vi "IETS_Tool_14_ProbeStation_SweepSaver.vi"() -> ()   [LabVIEW 2013]
doc: "I. Description:\nThis example demonstrates how to continuously acquire and generate data at the same time, synchronized with one another.\n\nII. Instructions for Running:\n1. Select the physical channel to correspond to where your signal is input on the DAQ device. Also, select the corresponding channel for where your signal is being generated.\n2. Enter the minimum and maximum voltage ranges.\nNote: For better accuracy try to match the input range to the expected voltage level of the measured signal.\n3. Set the sample rate of the acquisition.\nNote: The rate should be at least twice as fast as the maximum frequency component of the signal being acquired. \n6. Select the Rate for the generation\n7. Select what type of signal to generate and the amplitude.\nNote: This example requires two DMA channels to run. If your hardware does not support two DMA channels, you need to set the Data Transfer Mechanism property for the Analog Output Task to use \"Interrupts\". The Data Transfer Mechanism property is located in the DAQmx Channel Property hierarchy at:\n\nDAQmx Channel Property Node>>Analog Output>>General Properties>>Advanced>>Data Transfer and Memory>>Data Transfer Mechanism\n\nRefer to your device documentation to determine how many DMA channels are supported for your hardware.\n\nIII. Block Diagram Steps:\n1. Create an analog input voltage channel. Also, create an analog output voltage channel.\n2. Set the rate for the sample clock. Additionally, define the sample mode to be continuous. Also, set the sample clock rate for the signal generation.\n2a. Call the Get Terminal Name with Device Prefix VI. This will take a Task and a terminal and create a properly formatted device + terminal name to use as the source of the Trigger.\n3. Define the parameters for a Digital Edge Start Trigger. Set the Analog output to trigger off the AI Start Trigger. This is an internal trigger signal.\n4. Use the Basic Function Generator VI to create the signal to be generated.\n5. Call the Start VI to arm the two functions. Make sure the analog output is armed before the analog input. This will ensure both will start at the same time.\n6. Read the waveform data in a loop until the user hits the stop button or an error occurs. The Is Task Done? VI is used to check for errors in the Analog Output Task.\n7. Call the Clear VI to Clear the Task\n8. Use the popup dialog box to display an error if any.\n\nIV. I/O Connections Overview:\nMake sure your signal input/output terminals match the Physical Channel I/O controls."
uses:
  <vilib>/Utility/error.llb/DialogType.ctl
  <vilib>/DAQmx/write.llb/DAQmx Write (Analog 2D DBL NChan NSamp).vi
  <vilib>/DAQmx/read.llb/DAQmx Read (Analog 1D DBL NChan 1Samp).vi
  <vilib>/DAQmx/write.llb/DAQmx Write (Analog DBL 1Chan 1Samp).vi
  <vilib>/DAQmx/read.llb/DAQmx Read (Analog DBL 1Chan 1Samp).vi
  <vilib>/Analysis/baseanly.llb/Mean (DBL).vi
  <vilib>/DAQmx/write.llb/DAQmx Write (Analog 1D DBL NChan 1Samp).vi
  <vilib>/DAQmx/create/channels.llb/DAQmx Create Channel (AO-Voltage-Basic).vi
  <vilib>/DAQmx/create/channels.llb/DAQmx Create Channel (AI-Voltage-Basic).vi
  <vilib>/DAQmx/configure/timing.llb/DAQmx Timing (Sample Clock).vi
  <vilib>/DAQmx/configure/trigger.llb/DAQmx Start Trigger (Digital Edge).vi
  <vilib>/DAQmx/miscellaneous.llb/DAQmx Fill In Error Info.vi
  <vilib>/Utility/file.llb/Write To Spreadsheet File (DBL).vi
  pid/pid.llb/PID (DBL).vi
  pid/pid.llb/PID Output Rate Limiter (DBL).vi
  <vilib>/ptbypt/NI_PtbyPt.lvlib
  <resource>/objmgr/daqmx.rc
  <vilib>/Analysis/NI_AALBase.lvlib
panel:
  in  "Bias Offset Correct":dbl
  out "Bias Sweep":dbl[](graph)
  out "element":dbl
  out "mean":dbl format="%.6f"
  out "size(s)":i32
  out "Numeric":i32
  in  "PID":bool=TRUE caption="Step Z"
  in  "Tab Control":enum32{"PID Controller", "Tapping Controls"}(tab)=enum."Tapping Controls"
  in  "Proportional Gain":dbl=0.0001
  in  "Integral Gain":dbl=1e-07
  in  "Differential Gain":dbl=1e-05
  in  "Setpoint":dbl=0.1
  in  "Piezo Delta rate":dbl=1000.0
  in  "Min Current":dbl=0.002
  in  "Max Current":dbl=10.2
  in  "Ramp Rate":dbl=20.0
  in  "Make Contact":i32=1200
  in  "Break Contact":i32=500
  in  "Step Length":i32=100
  in  "Step Max":dbl=0.3
  in  "Step Min":dbl=0.05
  out "Tapping Stop":bool
  out "Case":i32
  in  "Contact Cycles":i32
  in  "Tapping":bool caption="Step Z"
  out "x/y":dbl
  out "Waveform Chart":dbl(graph)
  in  "Analog Ouyput 1":dbl(slide) min=-10.0 max=10.0 step=0.001 scale=-10.0..10.0
  in  "Manual Z":bool caption="Step Z"
  in  "Sweep Amplitude":dbl=1.0
  in  "Stop Sweep":bool
  out "Connections 2":string="AI0=Current\nAI1=Bias\nAI2=dI/dV\nAI3=d2I/dV2\nAI4=X-Axis\nAI5=Z-Axis\n"
  out "Connections":string="AO0=Bias\nAO1=Z-axis\nAO2=X-Axis\nAO3=NA"
  out "Save Indicator":bool
  in  "Z-Direction":bool caption="Step Z"
  in  "Update Bias":bool
  in  "Save Decay":bool
  in  "Step Z":bool
  in  "Comment":string="Molecule=TP4\nGain=10nA\nBias Gain=div/1\nSweep Freq.=0.0008Hz\nRef. Bias=4mV\nRef. Freq=2.977kHz\nGain LIA1=2mV\nTC LIA1=1s\nGain LIA2=5mV\nTC LIA2=1s\nLIA1=EGG\nLIA2=SRS\nEGG is driving(possible 5mV offset)"
  in  "Filenumber":i32
  in  "DATA Filename":string="Data_"
  in  "Data Directory":path=path "E:/Research/Data"
  out "Current Decay":cluster{dbl[], dbl[]}(graph)
  out "d2I/dV2":cluster{dbl[], dbl[]}(graph)
  out "dI/dV":cluster{dbl[], dbl[]}(graph)
  out "IV":cluster{dbl[], dbl[]}(graph)
  in  "# Samples":i32=2000
  in  "Frequency (Hz)":dbl=1.0
  out "Measurement 2":cluster{i32, dbl, dbl[]}(graph) caption="Measurement"
  out "Actual Update Generation Rate 2":dbl=5000.0 caption="Actual Update Generation Rate" format="%0.2f"
  in  "stop 3":bool
  in  "Bias":dbl=0.1 caption="Bias Start Point" step=0.1 format="%_3g"
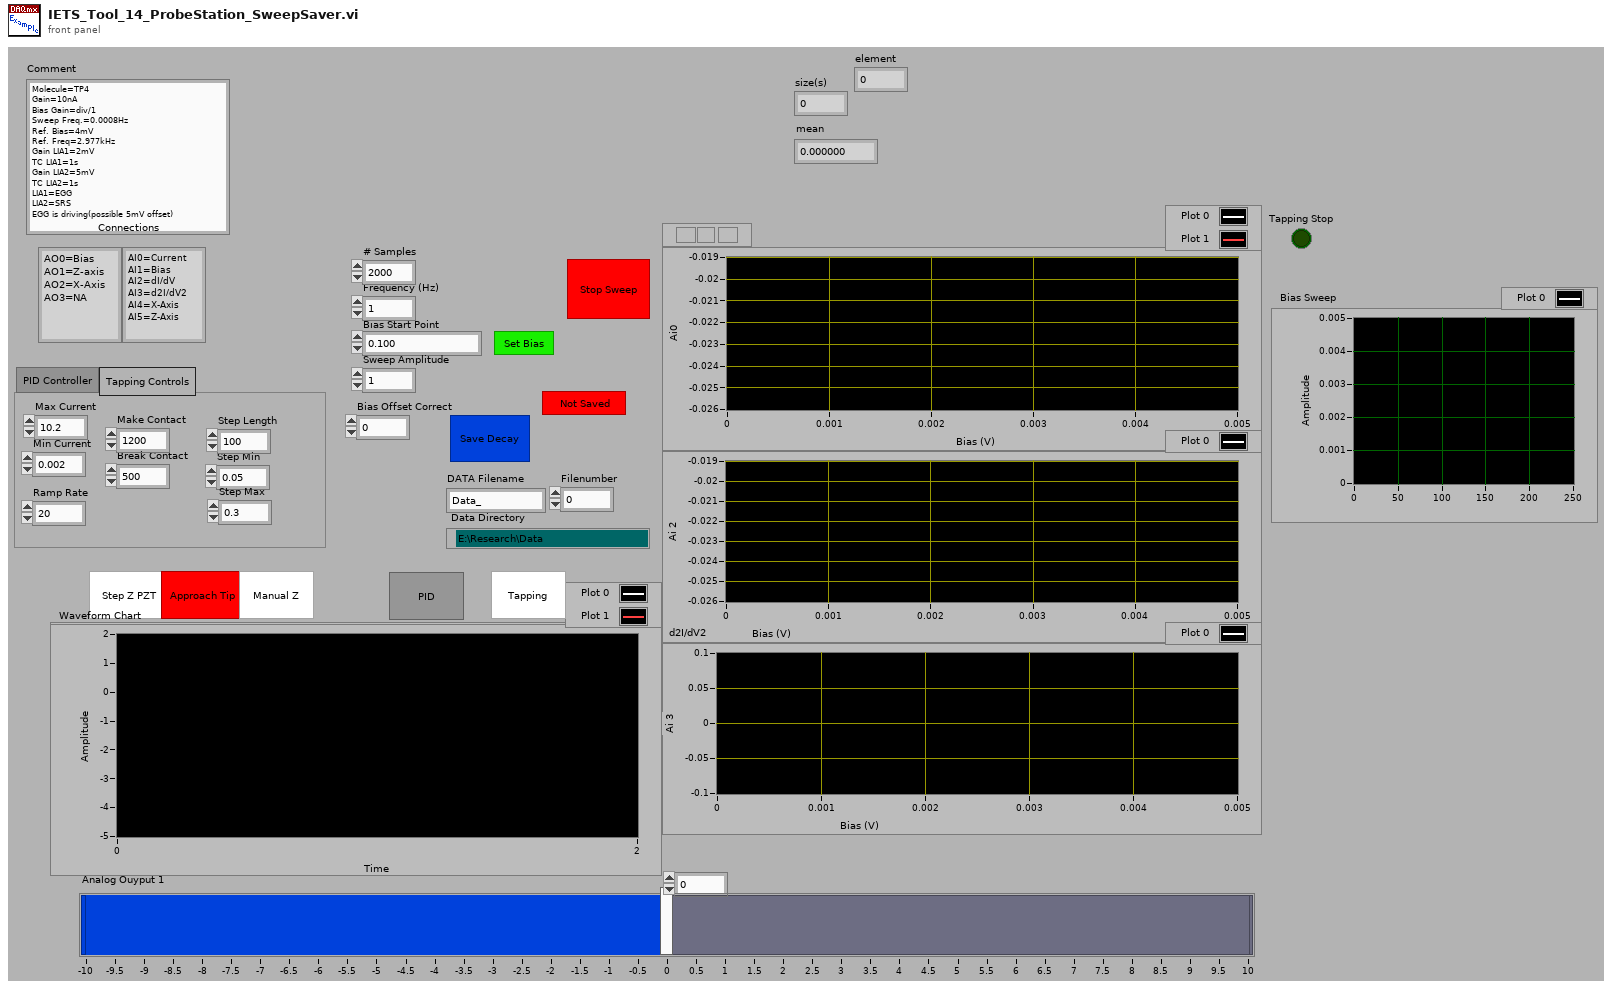
[diagram p1: front panel]
types:
  T1 = enum16{"open", "replace", "create", "open or create", "replace or create", "replace or create with confirmation"}
  T2 = typedef "DialogType.ctl" = u16
  T3 = cluster{"Proportional Gain":dbl, "Integral Gain ":dbl, "Differential Gain":dbl}
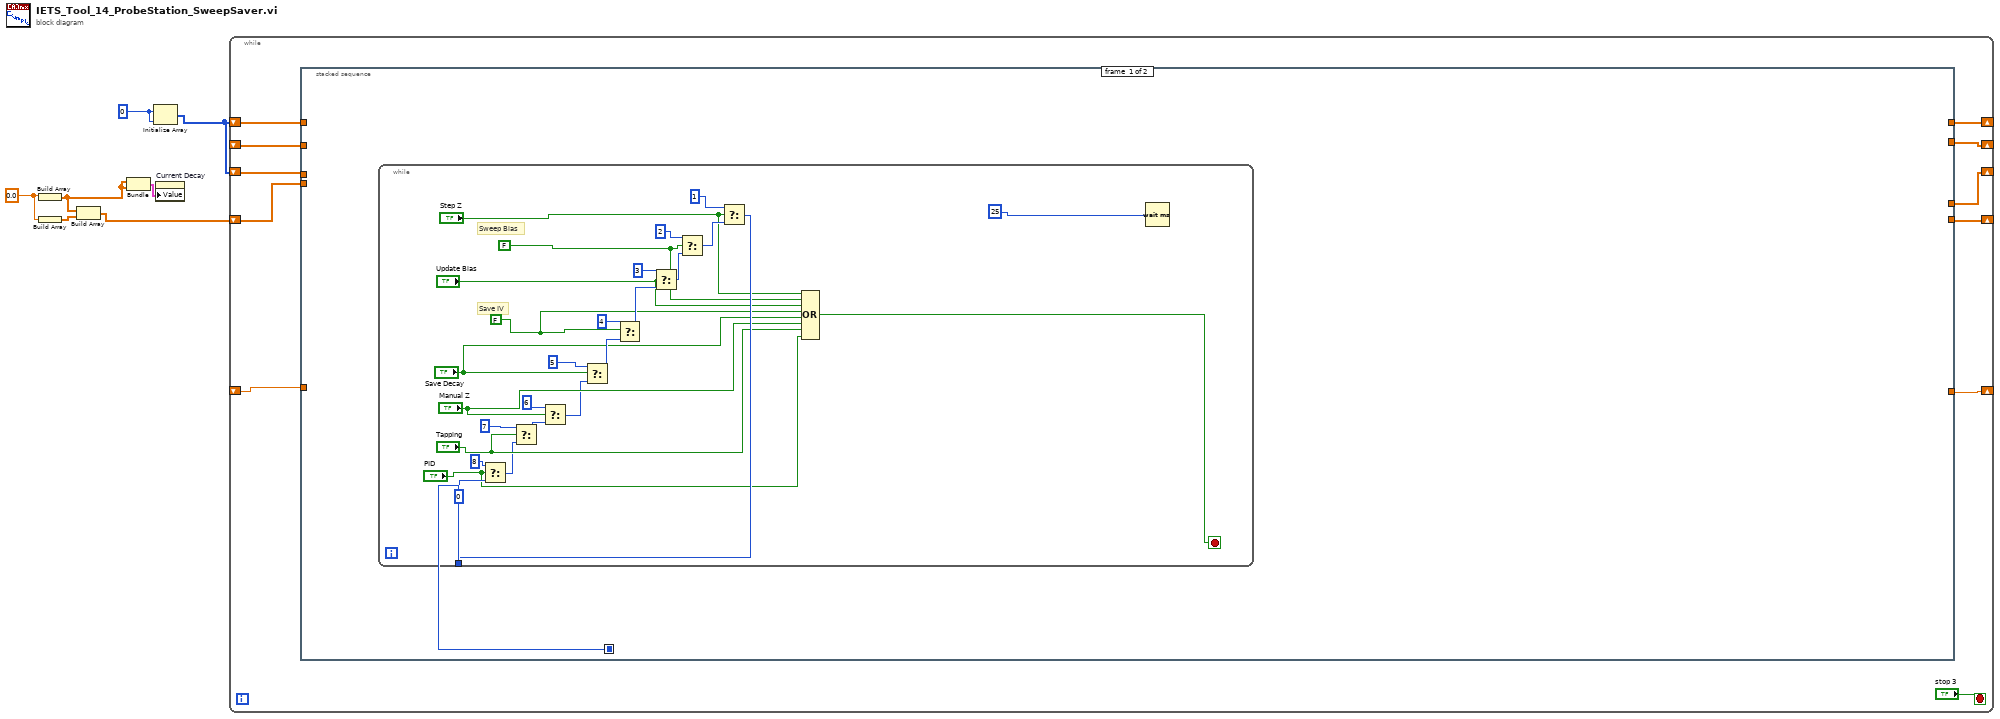
[diagram p0: block diagram]
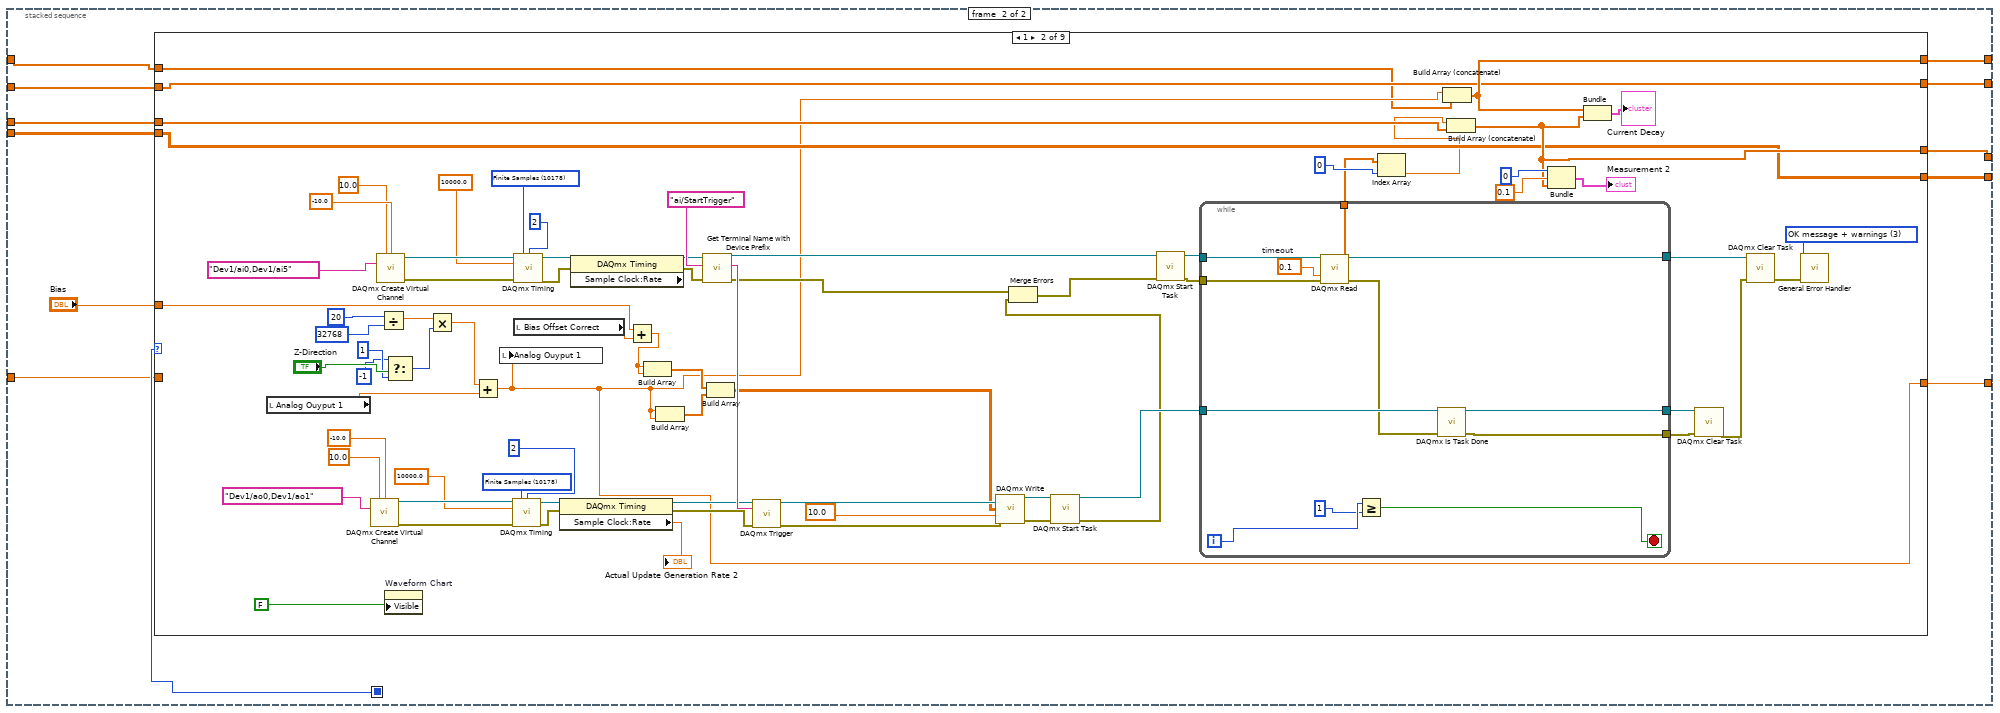
[diagram p2: hidden frame]
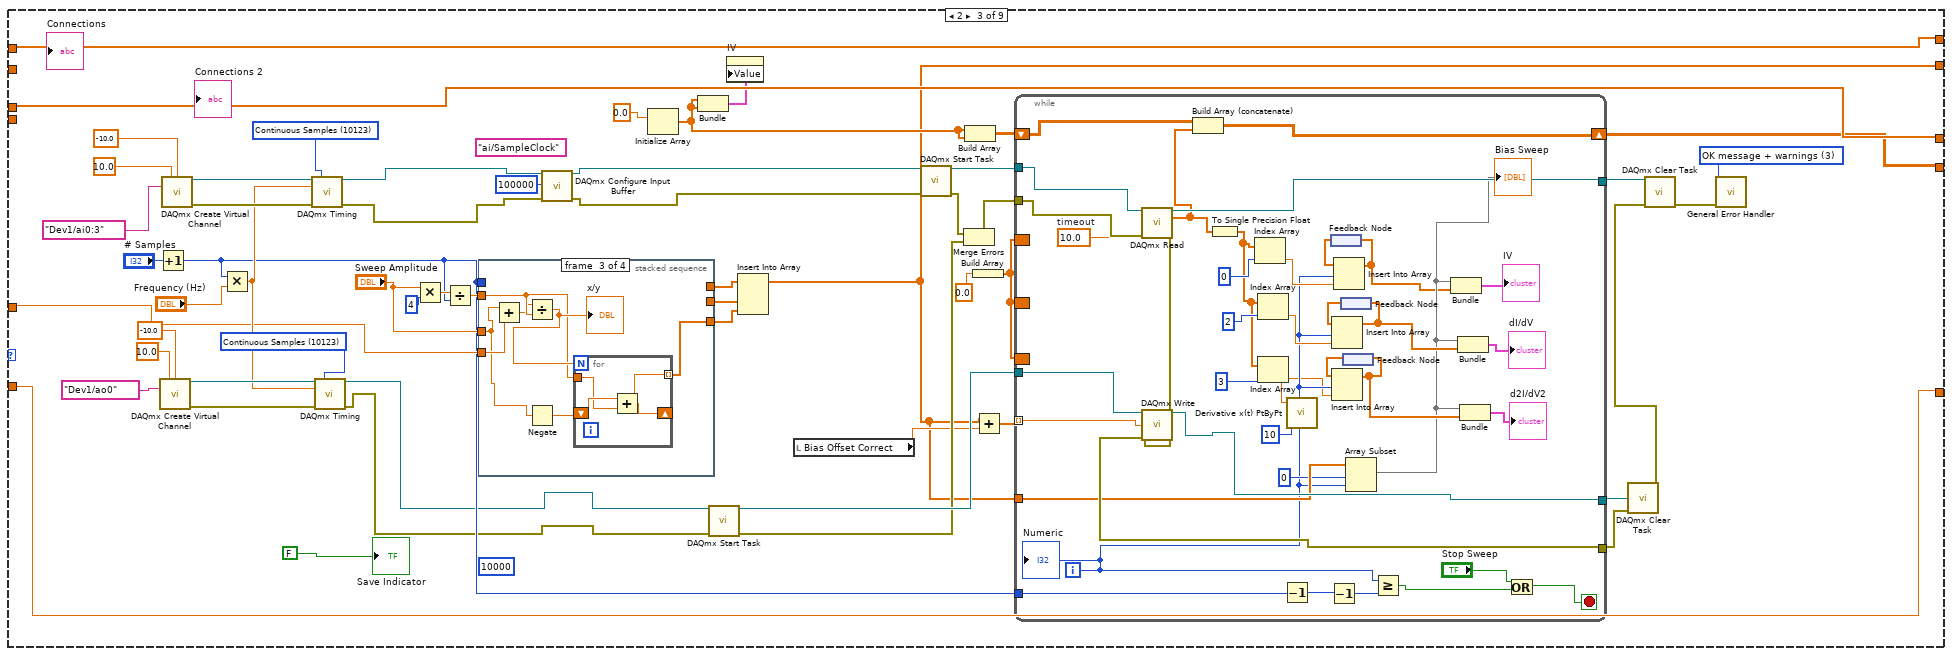
[diagram p4: hidden frame]
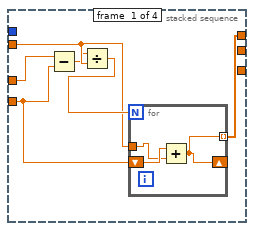
[diagram p5: hidden frame]
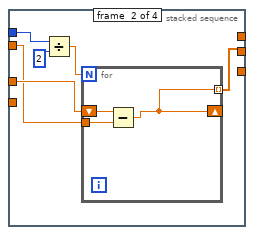
[diagram p6: hidden frame]
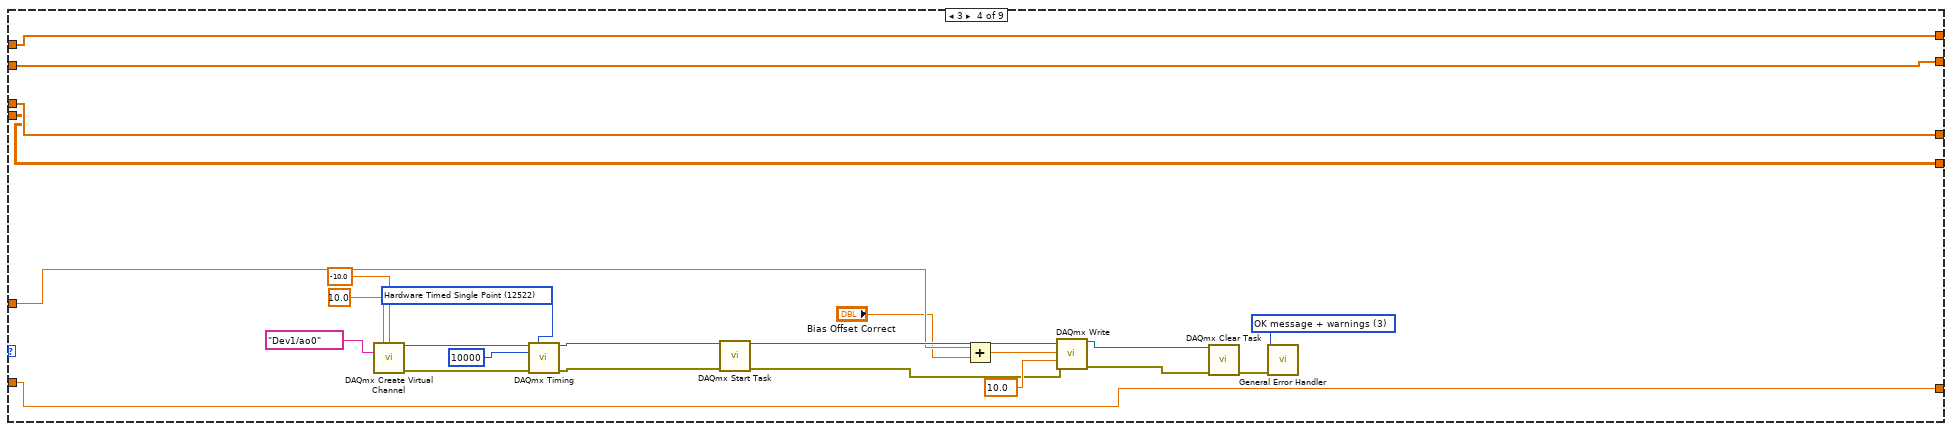
[diagram p8: hidden frame]
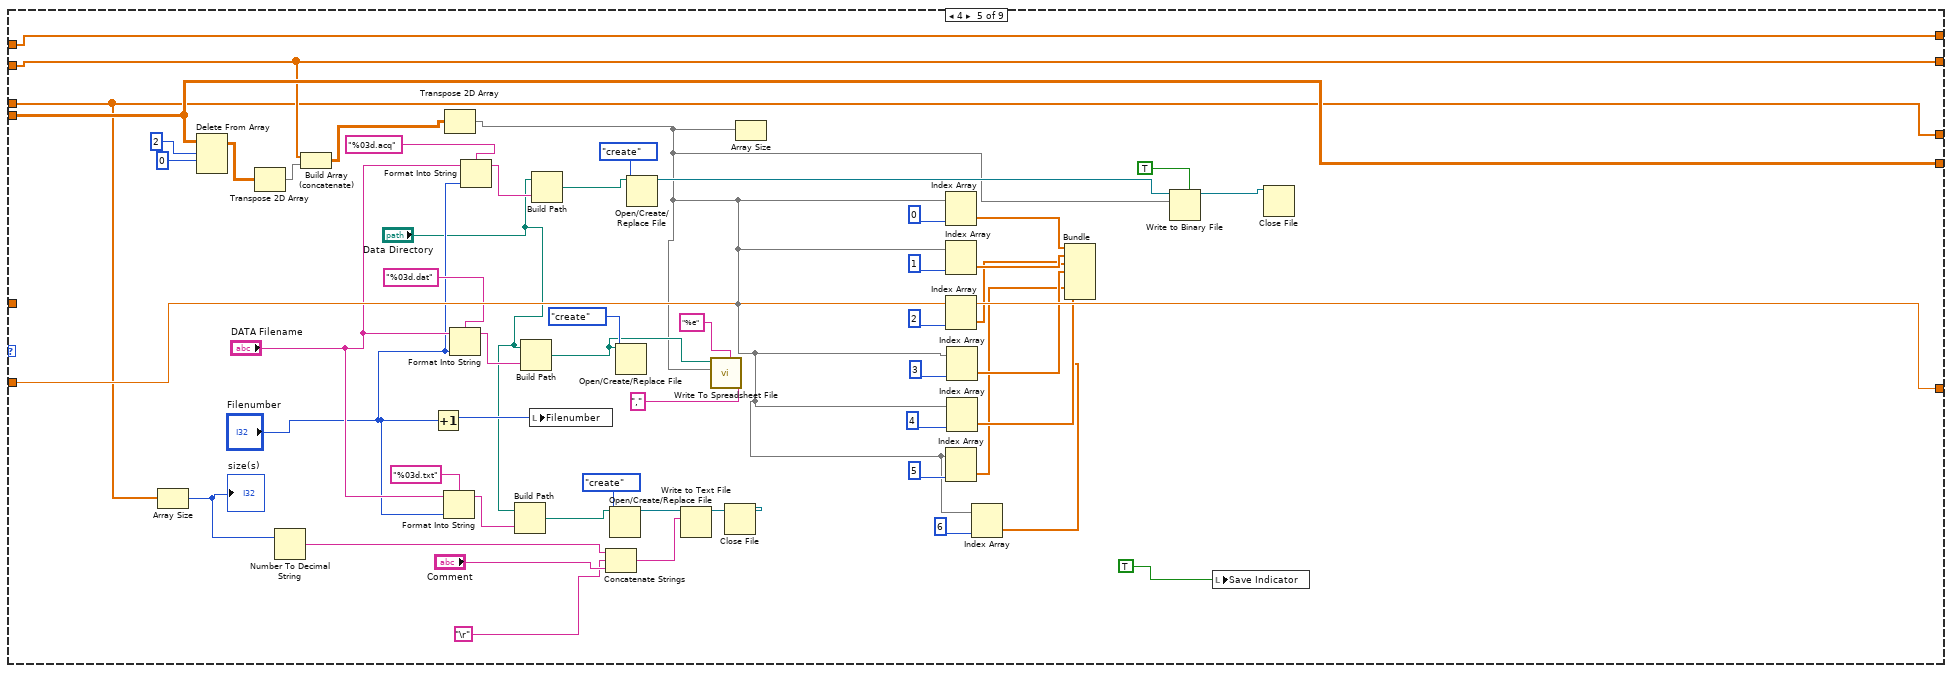
[diagram p9: hidden frame]
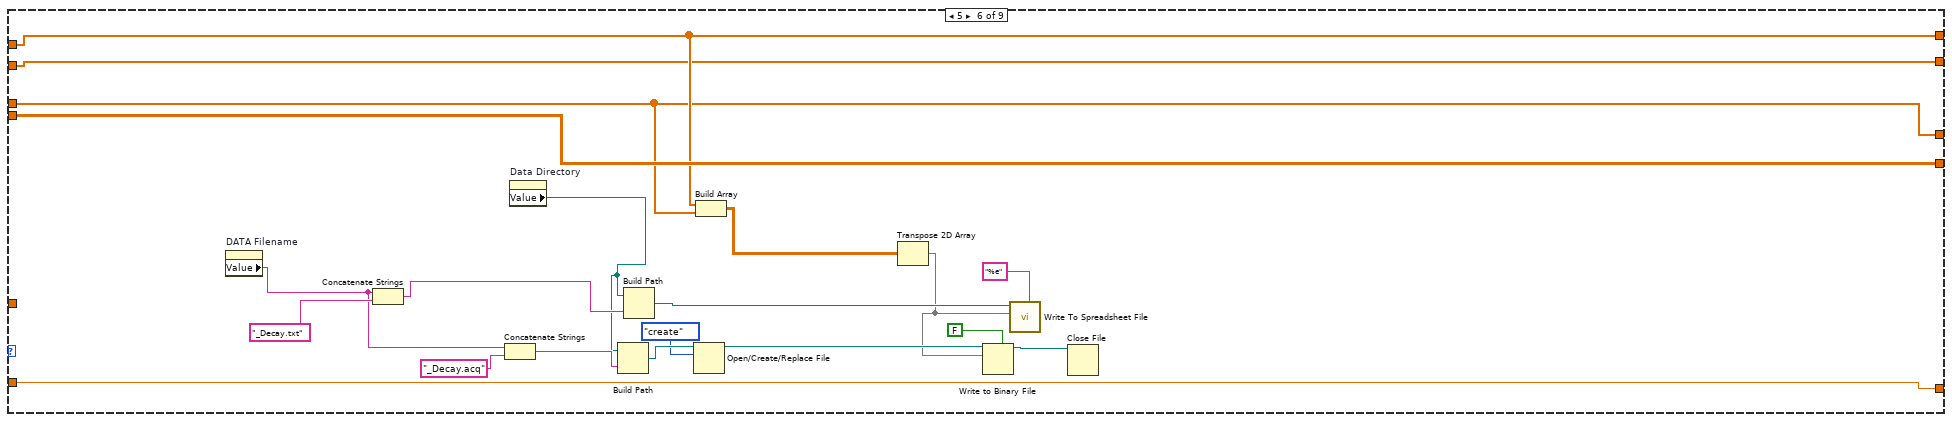
[diagram p10: hidden frame]
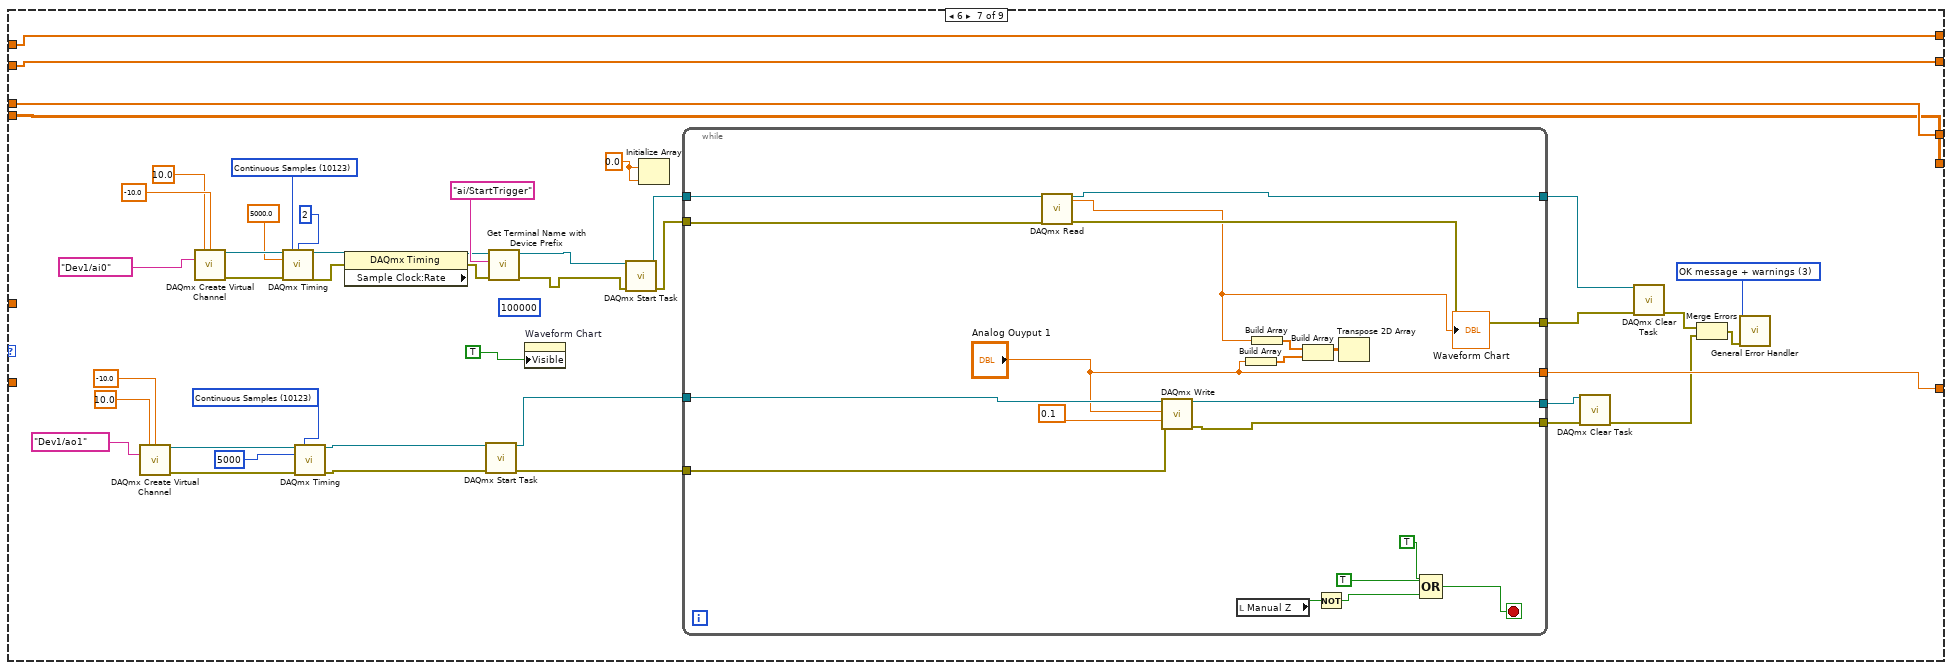
[diagram p11: hidden frame]
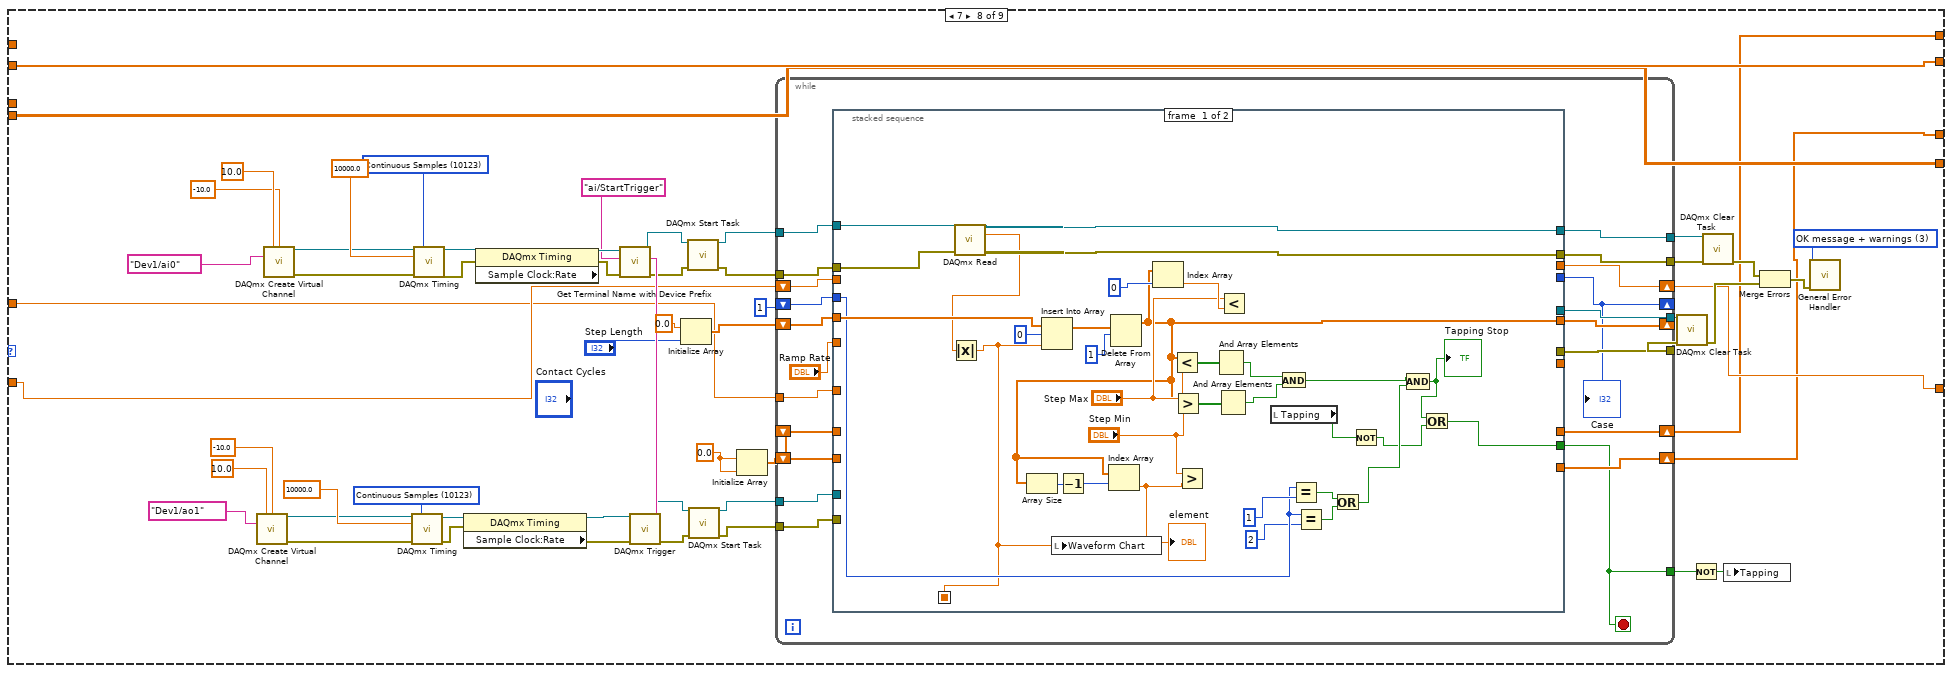
[diagram p12: hidden frame]
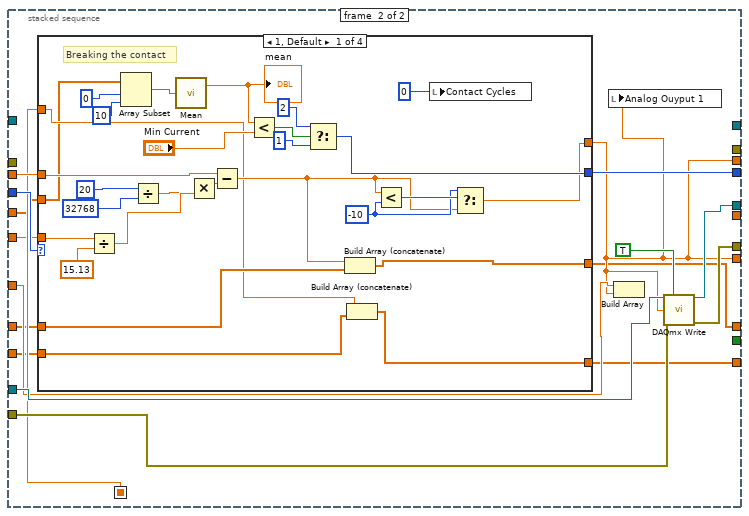
[diagram p13: hidden frame]
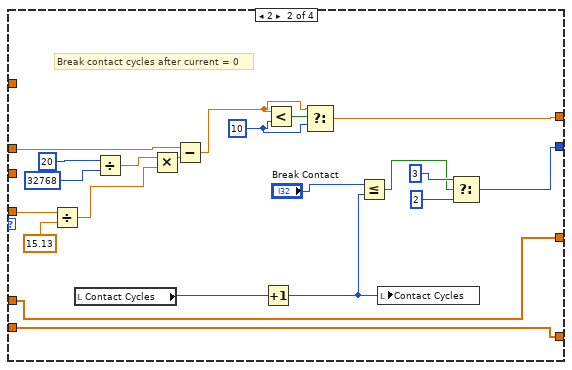
[diagram p14: hidden frame]
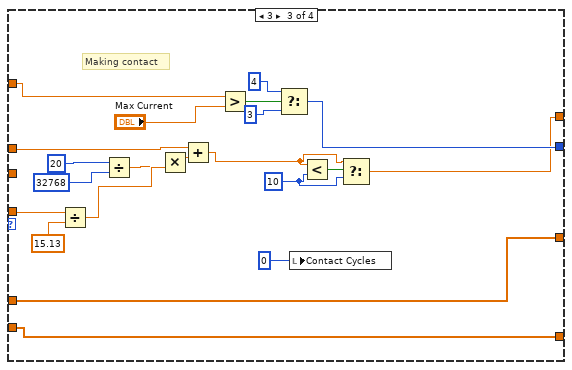
[diagram p15: hidden frame]
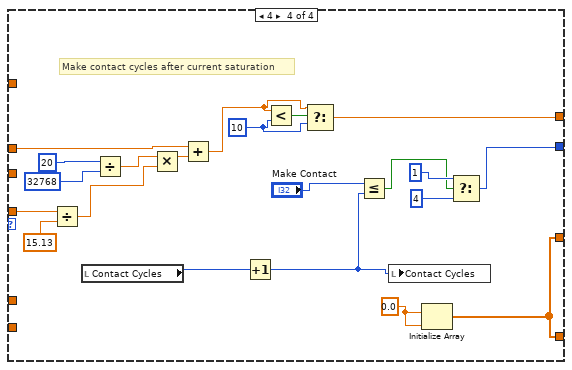
[diagram p16: hidden frame]
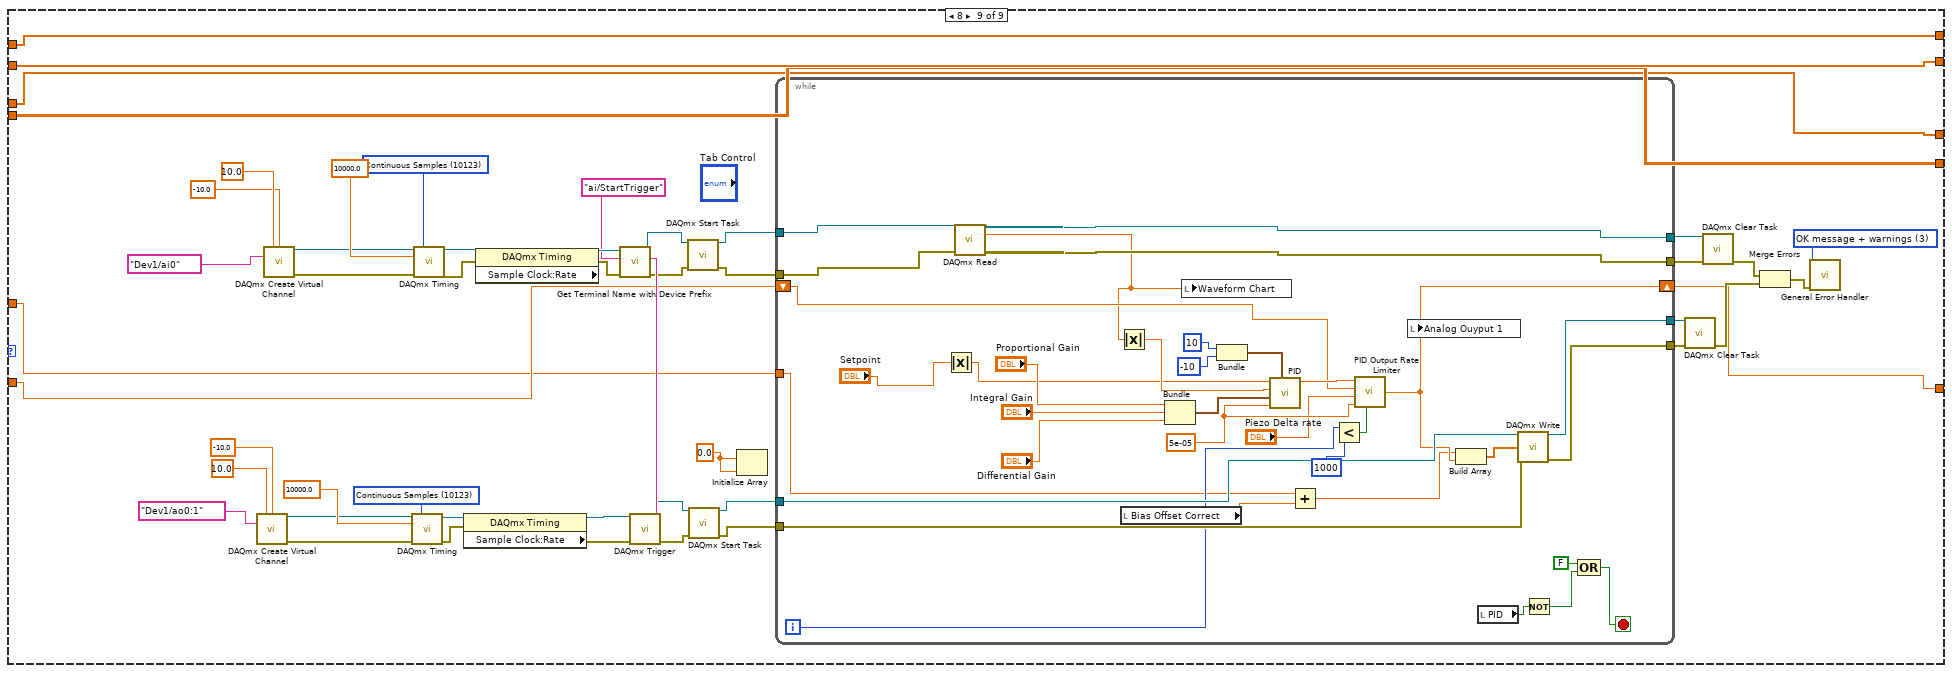
[diagram p17: hidden frame]
diagram:
  w2 = 0
  w7 = 0.0
  n1 = Build Array(w7) -> (w4:dbl[])
  n2 = Build Array(w7) -> (w6:dbl[])
  n3 = Build Array(w4, w6) -> (w5:dbl[][])
  n4 = Bundle(w4, w4) -> (w3:cluster{dbl[], dbl[]})  [unwired: 1 in]
  n5 = Initialize Array(w2, w2) -> (w1:i32[])
  n6 = property on="Current Decay" class="XYGraph (strict)"("Value"=w3) -> ()  [unwired: 2 in, 2 out]
  n7 = while {
    shift-right: [w16] -> _
    shift-left: w1 -> [w17]
    shift-right: [w14] -> _
    shift-left: w1 -> [w15]
    shift-right: [w12] -> _
    shift-left: _ -> [w13]
    shift-right: [w10] -> _
    shift-left: w5 -> [w11]
    shift-right: [w8] -> _
    shift-left: _ -> [w9]
    stop <- "stop 3" stop-if-true
    n8 = stacked-sequence {
      seq-local: [w19 _] -> [_ w58]
      tunnel: w17 -> [_ w57]
      tunnel: [_ w56] -> w16
      tunnel: w15 -> [_ w54]
      tunnel: [_ w53] -> w14
      tunnel: w13 -> [_ w52]
      tunnel: [_ w47] -> w12
      tunnel: w11 -> [_ w51]
      tunnel: [_ w50] -> w10
      tunnel: w9 -> [_ w49]
      tunnel: [_ w48] -> w8
      frame #0 {
        n9 = while {
          tunnel: [w37] -> w19
          stop <- w36 stop-if-true
          w20 = FALSE ("Sweep Bias")
          w21 = FALSE ("Save IV")
          # "Sweep Bias"
          # "Save IV"
          n10 = Select(t=8, s="PID", f=0) -> (s? t:f=w25:i32)
          n11 = Select(t=7, s="Tapping", f=w25) -> (s? t:f=w27:i32)
          n12 = Select(t=6, s="Manual Z", f=w27) -> (s? t:f=w28:i32)
          n13 = Select(t=5, s="Save Decay", f=w28) -> (s? t:f=w42:i32)
          n14 = Select(t=4, s=w21, f=w42) -> (s? t:f=w41:i32)
          n15 = Select(t=3, s="Update Bias", f=w41) -> (s? t:f=w39:i32)
          n16 = Select(t=2, s=w20, f=w39) -> (s? t:f=w46:i32)
          n17 = Select(t=1, s="Step Z", f=w46) -> (s? t:f=w37:i32)
          n18 = Compound Arithmetic op=OR("Step Z", w20, "Update Bias", w21, "Save Decay", "Manual Z", "Tapping", "PID") -> (w36:bool)
          n19 = Wait (ms)(milliseconds to wait=25) -> ()  [unwired: 1 out]
        }
      }
      frame #1 {
        n20 = case shown="1" w58 {
          tunnel: w57 -> [w63 w70 w190 w281 w301 w367 w412 _ w652]
          tunnel: [w63 w83 w190 w281 w301 w367 w412 w438 w652] -> w56
          tunnel: "Bias" -> [_ w66 w175 w275 _ _ _ w444 w651]
          tunnel: w54 -> [w62 w67 w187 w282 w347 w368 w414 _ w653]
          tunnel: [w62 w84 w187 w282 w347 w368 w414 w439 w653] -> w53
          tunnel: w52 -> [w61 _ w186 w280 w346 w369 _ w445 w660]
          tunnel: [w61 w68 w186 w280 w346 w369 w383 w440 w657] -> w47
          tunnel: w51 -> [w60 w81 _ w278 w326 w370 w411 w442 w658]
          tunnel: [w60 w81 w167 w278 w326 w370 w411 w442 w658] -> w50
          tunnel: [w59 w76 w151 w277 w324 w352 w413 w443 w659] -> w48
          tunnel: w49 -> [w59 w76 _ w277 w324 w352 w413 w443 w659]
          frame 0, Default {
          }
          frame 1 {
            w118 = T2 3 items=["no dialog", "OK message", "continue or stop message", "OK message + warnings", "continue/stop + warnings"] ("type of dialog (OK msg:1)")
            w130 = 10178 items=["Finite Samples"=10178, "Continuous Samples"=10123] ("sample mode")
            w135 = 10178 items=["Finite Samples"=10178, "Continuous Samples"=10123] ("sample mode")
            n21 = local read "Analog Ouyput 1"() -> (w71:dbl)
            n22 = call-poly <vilib>:"DAQmx Create Virtual Channel.vi"("maximum value"=10.0 ("maximum value 2"), "minimum value"=-10.0 ("minimum value 2"), "physical channels"=tag "Dev1/ao0,Dev1/ao1" ("physical channels 2")) -> ("task out"=w129:refnum<k21>, "error out"=w128:errorcluster)  [unwired: 11 in]
            n23 = call-poly <vilib>:"DAQmx Create Virtual Channel.vi"("maximum value"=10.0 ("Maximum Value 2"), "minimum value"=-10.0 ("Minimum Value 2"), "physical channels"=tag "Dev1/ai0,Dev1/ai5" ("Physical Channel 2")) -> ("task out"=w133:refnum<k21>, "error out"=w134:errorcluster)  [unwired: 11 in]
            n24 = Divide(x=20, y=32768) -> (x/y=w80:dbl)
            n25 = property on="Waveform Chart" class="WFChart (strict)"("Visible"=FALSE) -> ()  [unwired: 2 in, 2 out]
            n26 = Select(t=-1 ("f"), s="Z-Direction", f=1) -> (s? t:f=w78:i32)
            n27 = Multiply(x=w80, y=w78) -> (x*y=w79:dbl)
            n28 = Add(x=w79, y=w71) -> (x+y=w68:dbl)
            n29 = local write "Analog Ouyput 1"(w68) -> ()
            n30 = call-poly <vilib>:"DAQmx Timing.vi"("task/channels in"=w129, "sample mode"=w130, "samples per channel"=2, "rate"=10000.0 ("rate 2"), "error in"=w128) -> ("task out"=w113:refnum<k21>, "error out"=w112:errorcluster)  [unwired: 9 in]
            n31 = call-poly <vilib>:"DAQmx Timing.vi"("task/channels in"=w133, "sample mode"=w135, "samples per channel"=2, "rate"=10000.0 ("Rate 2"), "error in"=w134) -> ("task out"=w107:refnum<k21>, "error out"=w106:errorcluster)  [unwired: 9 in]
            n32 = local read "Bias Offset Correct"() -> (w65:dbl)
            n33 = property class="DAQmx Timing"(reference=w113, error in=w112) -> (reference out=w114:refnum<k21>, error out=w111:errorcluster, "Sample Clock:Rate"=→"Actual Update Generation Rate 2":dbl)
            n34 = property class="DAQmx Timing" props=["Sample Clock:Rate"](reference=w107, error in=w106) -> (reference out=w105:refnum<k21>, error out=w104:errorcluster)  [unwired: 1 out]
            n35 = Add(x=w66, y=w65) -> (x+y=w64:dbl)
            n36 = Build Array(w64, w64) -> (w91:dbl[])
            n37 = Build Array(w68, w68) -> (w90:dbl[])
            n38 = call "Get Terminal Name with Device Prefix.vi"("error in (no error)"=w104, "Local Terminal Name"="ai/StartTrigger" ("terminal"), "task/channels in"=w105) -> ("error out"=w110:errorcluster, "Terminal Name with Device Prefix"=w115:tag, "task out"=w95:refnum<k21>)  [unwired: 6 in]
            n39 = Build Array(w91, w90) -> (w89:dbl[][])
            n40 = call-poly <vilib>:"DAQmx Trigger.vi"("task/channels in"=w114, "source"=w115, "error in"=w111) -> ("task out"=w120:refnum<k21>, "error out"=w121:errorcluster)  [unwired: 11 in]
            n41 = call-poly <vilib>:"DAQmx Write.vi"("task/channels in"=w120, "data"=w89, "timeout"=10.0 ("Wirite Timeout"), "error in"=w121) -> ("task out"=w123:refnum<k21>, "error out"=w122:errorcluster)  [unwired: 9 in, 1 out]
            n42 = call <vilib>:"DAQmx Start Task.vi"("task/channels in"=w123, "error in"=w122) -> ("task out"=w127:refnum<k21>, "error out"=w109:errorcluster)  [unwired: 12 in]
            n43 = Merge Errors(w110, w109) -> (w97:errorcluster)
            n44 = call <vilib>:"DAQmx Start Task.vi"("task/channels in"=w95, "error in"=w97) -> ("task out"=w94:refnum<k21>, "error out"=w96:errorcluster)  [unwired: 12 in]
            n45 = while {
              tunnel: [w150] -> w136
              tunnel: w127 -> [w149]
              tunnel: [w148] -> w126
              tunnel: w94 -> [w139]
              tunnel: [w147] -> w103
              tunnel: [w144] -> w87
              tunnel: w96 -> [w140]
              i -> [w143]
              stop <- w141 stop-if-true
              w146 = 0.1  # timeout
              n46 = call-poly <vilib>:"DAQmx Read.vi"("task/channels in"=w139, "timeout"=w146, "error in"=w140) -> ("task out"=w150:refnum<k21>, "data"=w144:dbl[], "error out"=w145:errorcluster)  [unwired: 10 in]
              n47 = Greater Or Equal?(x=w143, y=1) -> (x >= y?=w141:bool)
              n48 = call <vilib>:"DAQmx Is Task Done.vi"("task/channels in"=w149, "error in"=w145) -> ("task out"=w148:refnum<k21>, "error out"=w147:errorcluster)  [unwired: 11 in, 1 out]
            }
            n49 = Index Array(array=w87, index=0) -> (element=w69:dbl)
            n50 = Build Array (concatenate)(w68, w67) -> (w84:dbl[])
            n51 = Build Array (concatenate)(w69, w70) -> (w83:dbl[])
            n52 = Bundle(0, 0.1, w83) -> (→"Measurement 2":cluster{i32, dbl, dbl[]})  [unwired: 1 in]
            n53 = Bundle(w84, w83) -> (→"Current Decay":cluster{dbl[], dbl[]})  [unwired: 1 in]
            n54 = call <vilib>:"DAQmx Clear Task.vi"("task in"=w126, "error in"=w103) -> ("error out"=w102:errorcluster)  [unwired: 13 in]
            n55 = call <vilib>:"DAQmx Clear Task.vi"("task in"=w136, "error in"=w102) -> ("error out"=w101:errorcluster)  [unwired: 13 in]
            n56 = call <vilib>:"General Error Handler.vi"("type of dialog (OK msg:1)"=w118, "error in (no error)"=w101) -> ()  [unwired: 9 in, 5 out]
          }
          frame 2 {
            (unwired) 10000
            w184 = 10123 items=["Finite Samples"=10178, "Continuous Samples"=10123, "Hardware Timed Single Point"=12522] ("sample mode")
            w185 = 10123 items=["Finite Samples"=10178, "Continuous Samples"=10123, "Hardware Timed Single Point"=12522] ("sample mode")
            (unwired) "ai/SampleClock" ("terminal")
            w195 = T2 3 items=["no dialog", "OK message", "continue or stop message", "OK message + warnings", "continue/stop + warnings"] ("type of dialog (OK msg:1)")
            n57 = Increment(x="# Samples") -> (x+1=w165:i32)
            n58 = call-poly <vilib>:"DAQmx Create Virtual Channel.vi"("maximum value"=10.0, "minimum value"=-10.0, "physical channels"=tag "Dev1/ao0") -> ("task out"=w198:refnum<k21>, "error out"=w197:errorcluster)  [unwired: 11 in]
            n59 = call-poly <vilib>:"DAQmx Create Virtual Channel.vi"("maximum value"=10.0 ("Maximum Value"), "minimum value"=-10.0 ("Minimum Value"), "physical channels"=tag "Dev1/ai0:3" ("Physical Channel")) -> ("task out"=w202:refnum<k21>, "error out"=w203:errorcluster)  [unwired: 11 in]
            n60 = Multiply(x=w165, y="Frequency (Hz)") -> (x*y=w189:dbl)
            n61 = call-poly <vilib>:"DAQmx Timing.vi"("task/channels in"=w202, "sample mode"=w184, "rate"=w189, "error in"=w203) -> ("task out"=w160:refnum<k21>, "error out"=w158:errorcluster)  [unwired: 10 in]
            n62 = call-poly <vilib>:"DAQmx Timing.vi"("task/channels in"=w198, "sample mode"=w185, "rate"=w189, "error in"=w197) -> ("task out"=w155:refnum<k21>, "error out"=w154:errorcluster)  [unwired: 10 in]
            n63 = Multiply(x="Sweep Amplitude", y=4) -> (x*y=w173:dbl)
            n64 = Divide(x=w173, y=w165) -> (x/y=w172:dbl)
            n65 = stacked-sequence {
              tunnel: "Sweep Amplitude" -> [w251 w257 w265 _]
              tunnel: w175 -> [w249 _ w269 _]
              tunnel: w172 -> [w247 w256 w267 _]
              tunnel: [w248 _ _ _] -> w171
              tunnel: w165 -> [_ w260 _ _]
              tunnel: [_ w255 _ _] -> w170
              tunnel: [_ _ w268 _] -> w169
              frame #0 {
                n66 = Subtract(x=w251, y=w249) -> (x-y=w246:dbl)
                n67 = Divide(x=w246, y=w247) -> (x/y=w250:dbl)
                n68 = for {
                  N: w250 -> [_]
                  tunnel: w247 -> [w253]
                  shift-right: [w252] -> _
                  shift-left: w249 -> [w254]
                  tunnel: [w252] -> w248 mode=indexing
                  n69 = Add(x=w254, y=w253) -> (x+y=w252:dbl)
                }
              }
              frame #1 {
                n70 = Divide(x=w260, y=2) -> (x/y=w258:dbl)
                n71 = for {
                  N: w258 -> [_]
                  tunnel: w256 -> [w262]
                  shift-right: [w261] -> _
                  shift-left: w257 -> [w263]
                  tunnel: [w261] -> w255 mode=indexing
                  n72 = Subtract(x=w263, y=w262) -> (x-y=w261:dbl)
                }
              }
              frame #2 {
                n73 = Add(x=w265, y=w269) -> (x+y=w266:dbl)
                n74 = Divide(x=w266, y=w267) -> (x/y=w270:dbl)
                "x/y" <- w270
                n75 = Negate(x=w265) -> (-x=w264:dbl)
                n76 = for {
                  N: w270 -> [_]
                  tunnel: w267 -> [w272]
                  shift-right: [w271] -> _
                  shift-left: w264 -> [w273]
                  tunnel: [w271] -> w268 mode=indexing
                  n77 = Add(x=w273, y=w272) -> (x+y=w271:dbl)
                }
              }
              frame #3 {
              }
            }
            n78 = call <vilib>:"DAQmx Configure Input Buffer.vi"("task/channels in"=w160, "buffer size (in samples per channel)"=100000, "error in"=w158) -> ("task out"=w159:refnum<k21>, "error out"=w157:errorcluster)  [unwired: 11 in]
            n79 = Initialize Array(0.0) -> (w164:dbl[])  [unwired: 1 in]
            n80 = Bundle(w164, w164) -> (w163:cluster{dbl[], dbl[]})  [unwired: 1 in]
            n81 = call <vilib>:"DAQmx Start Task.vi"("task/channels in"=w155, "error in"=w154) -> ("task out"=w183:refnum<k21>, "error out"=w179:errorcluster)  [unwired: 12 in]
            n82 = property on="IV" class="XYGraph (strict)"("Value"=w163) -> ()  [unwired: 2 in, 2 out]
            n83 = Insert Into Array(array=w171, new element #1=w170, new element #2=w169) -> (w151:dbl[])  [unwired: 1 in]
            n84 = local read "Bias Offset Correct"() -> (w152:dbl)
            n85 = call <vilib>:"DAQmx Start Task.vi"("task/channels in"=w159, "error in"=w157) -> ("task out"=w181:refnum<k21>, "error out"=w180:errorcluster)  [unwired: 12 in]
            n86 = Merge Errors(w180, w179) -> (w182:errorcluster)
            n87 = Build Array(w164, w164) -> (w166:dbl[][])
            n88 = Build Array(0.0) -> (w161:dbl[])
            n89 = Add(x=w151, y=w152) -> (x+y=w153:dbl[])
            n90 = while {
              tunnel: [w237] -> w204
              tunnel: [w240] -> w196
              tunnel: [w239] -> w193
              tunnel: w165 -> [w213]
              tunnel: w153 -> [w218] mode=indexing
              tunnel: w183 -> [w242]
              tunnel: w181 -> [w245]
              tunnel: w182 -> [w244]
              shift-right: [w219] -> w167
              shift-left: w166 -> [w238]
              tunnel: w151 -> [w235]
              border: w161 -> [_]
              border: w161 -> [_]
              border: w161 -> [_]
              i -> [w214]
              stop <- w215 stop-if-true
              w241 = 10.0  # timeout
              n91 = call-poly <vilib>:"DAQmx Read.vi"("task/channels in"=w245, "timeout"=w241, "error in"=w244) -> ("task out"=w237:refnum<k21>, "data"=w221:dbl[], "error out"=w243:errorcluster)  [unwired: 10 in]
              n92 = call-poly <vilib>:"DAQmx Write.vi"("task/channels in"=w242, "data"=w218, "error in"=w243) -> ("task out"=w240:refnum<k21>, "error out"=w239:errorcluster)  [unwired: 10 in, 1 out]
              n93 = Build Array (concatenate)(w238, w221) -> (w219:dbl[][])
              n94 = To Single Precision Float(number=w221) -> (single precision float=w220:sgl[])
              n95 = Index Array(array=w220, index=0) -> (element=w233:sgl)
              n96 = Index Array(array=w220, index=2) -> (element=w229:sgl)
              n97 = Index Array(array=w220, index=3) -> (element=w209:sgl)
              n98 = Decrement(x=w213) -> (x-1=w211:i32)
              n99 = call <vilib>:"Derivative x(t) PtByPt.vi"("dt"=10, "x"=w209) -> ()  [unwired: 2 in, 2 out]
              n100 = Decrement(x=w211) -> (x-1=w212:i32)
              n101 = feedback #1() -> (w232:dbl[])
              n102 = Insert Into Array(array=w232, index=w214, new element=w233) -> (w207:dbl[])
              n103 = feedback-in #1(w207) -> ()
              n104 = feedback #2() -> (w228:dbl[])
              n105 = Insert Into Array(array=w228, index=w214, new element=w229) -> (w226:dbl[])
              n106 = feedback-in #2(w226) -> ()
              n107 = feedback #3() -> (w227:dbl[])
              n108 = Insert Into Array(array=w227, index=w214, new element=w209) -> (w225:dbl[])
              n109 = feedback-in #3(w225) -> ()
              n110 = Array Subset(array=w235, index=0, length=w214) -> (w208:dbl[])
              "Bias Sweep" <- w208
              n111 = Greater Or Equal?(x=w214, y=w212) -> (x >= y?=w216:bool)
              n112 = Bundle(w208, w207) -> (→"IV":cluster{dbl[], dbl[]})  [unwired: 1 in]
              n113 = Bundle(w208, w226) -> (→"dI/dV":cluster{dbl[], dbl[]})  [unwired: 1 in]
              n114 = Bundle(w208, w225) -> (→"d2I/dV2":cluster{dbl[], dbl[]})  [unwired: 1 in]
              n115 = Or(x="Stop Sweep", y=w216) -> (x .or. y?=w215:bool)
              "Numeric" <- w214
            }
            n116 = call <vilib>:"DAQmx Clear Task.vi"("task in"=w196, "error in"=w193) -> ("error out"=w192:errorcluster)  [unwired: 13 in]
            n117 = call <vilib>:"DAQmx Clear Task.vi"("task in"=w204, "error in"=w192) -> ("error out"=w191:errorcluster)  [unwired: 13 in]
            n118 = call <vilib>:"General Error Handler.vi"("type of dialog (OK msg:1)"=w195, "error in (no error)"=w191) -> ()  [unwired: 9 in, 5 out]
            "Save Indicator" <- FALSE
          }
          frame 3 {
            w286 = T2 3 items=["no dialog", "OK message", "continue or stop message", "OK message + warnings", "continue/stop + warnings"] ("type of dialog (OK msg:1)")
            w291 = 12522 items=["Finite Samples"=10178, "Continuous Samples"=10123, "Hardware Timed Single Point"=12522] ("sample mode")
            n119 = call-poly <vilib>:"DAQmx Create Virtual Channel.vi"("maximum value"=10.0 ("maximum value 2"), "minimum value"=-10.0 ("minimum value 2"), "physical channels"=tag "Dev1/ao0" ("physical channels 2")) -> ("task out"=w294:refnum<k21>, "error out"=w293:errorcluster)  [unwired: 11 in]
            n120 = call-poly <vilib>:"DAQmx Timing.vi"("task/channels in"=w294, "sample mode"=w291, "rate"=10000, "error in"=w293) -> ("task out"=w290:refnum<k21>, "error out"=w289:errorcluster)  [unwired: 10 in]
            n121 = call <vilib>:"DAQmx Start Task.vi"("task/channels in"=w290, "error in"=w289) -> ("task out"=w288:refnum<k21>, "error out"=w287:errorcluster)  [unwired: 12 in]
            n122 = Add(x=w275, y="Bias Offset Correct") -> (x+y=w276:dbl)
            n123 = call-poly <vilib>:"DAQmx Write.vi"("task/channels in"=w288, "data"=w276, "timeout"=10.0 ("Wirite Timeout"), "error in"=w287) -> ("task out"=w284:refnum<k21>, "error out"=w283:errorcluster)  [unwired: 9 in, 1 out]
            n124 = call <vilib>:"DAQmx Clear Task.vi"("task in"=w284, "error in"=w283) -> ("error out"=w285:errorcluster)  [unwired: 13 in]
            n125 = call <vilib>:"General Error Handler.vi"("type of dialog (OK msg:1)"=w286, "error in (no error)"=w285) -> ()  [unwired: 9 in, 5 out]
          }
          frame 4 {
            n126 = Array Size(array=w301) -> (size(s)=w300:i32)
            "size(s)" <- w300
            n127 = Delete From Array(array=w326, length=2, index (row)=0) -> (array with subset deleted=w323:dbl[][])  [unwired: 1 in, 1 out]
            n128 = Transpose 2D Array(2D array=w323) -> (transposed array=w322:dbl[][])
            n129 = Number To Decimal String(number=w300) -> (decimal integer string=w299:string)  [unwired: 1 in]
            n130 = Build Array (concatenate)(w324, w322) -> (w305:dbl[][])
            n131 = Increment(x="Filenumber") -> (x+1=w349:i32)
            n132 = Format Into String(format string="%03d.txt", initial string="DATA Filename", "Filenumber") -> (resulting string=w337:string)  [unwired: 1 in, 1 out]
            n133 = Transpose 2D Array(2D array=w305) -> (transposed array=w304:dbl[][])
            n134 = Format Into String(format string="%03d.dat", initial string="DATA Filename", "Filenumber") -> (resulting string=w351:string)  [unwired: 1 in, 1 out]
            n135 = Format Into String(format string="%03d.acq", initial string="DATA Filename", "Filenumber") -> (resulting string=w344:string)  [unwired: 1 in, 1 out]
            n136 = Build Path(base path="Data Directory", name or relative path=w337) -> (appended path=w335:path)
            n137 = Build Path(base path="Data Directory", name or relative path=w351) -> (appended path=w348:path)
            n138 = local write "Filenumber"(w349) -> ()
            n139 = Build Path(base path="Data Directory", name or relative path=w344) -> (appended path=w342:path)
            n140 = Concatenate Strings(w299, "\r", "Comment") -> (w320:string)
            n141 = Open/Create/Replace File(file path (use dialog)=w335, operation (0:open)=T1."create") -> (refnum out=w330:refnum<file>)  [unwired: 4 in, 2 out]
            n142 = Open/Create/Replace File(file path (use dialog)=w348, operation (0:open)=T1."create") -> ()  [unwired: 4 in, 3 out]
            n143 = Open/Create/Replace File(file path (use dialog)=w342, operation (0:open)=T1."create") -> (refnum out=w341:refnum<file>)  [unwired: 4 in, 2 out]
            n144 = Write to Text File(file (use dialog)=w330, text=w320) -> (refnum out=w329:refnum<file>)  [unwired: 2 in, 2 out]
            n145 = call-poly <vilib>:"Write To Spreadsheet File.vi"("delimiter (\\t)"=",", "format (%.3f)"="%e", "2D data"=w304, "file path (dialog if empty)"=w348) -> ()  [unwired: 4 in, 1 out]
            n146 = Close File(refnum=w329) -> ()  [unwired: 1 in, 2 out]
            n147 = Array Size(array=w304) -> ()  [unwired: 1 out]
            n148 = Index Array(array=w304, index (col)=0) -> (element=w312:dbl[])  [unwired: 1 in]
            n149 = Index Array(array=w304, index (col)=1) -> (element=w311:dbl[])  [unwired: 1 in]
            n150 = Index Array(array=w304, index (col)=2) -> (element=w310:dbl[])  [unwired: 1 in]
            n151 = Index Array(array=w304, index (col)=5) -> (element=w307:dbl[])  [unwired: 1 in]
            n152 = Index Array(array=w304, index (col)=3) -> (element=w309:dbl[])  [unwired: 1 in]
            n153 = Index Array(array=w304, index (col)=4) -> (element=w308:dbl[])  [unwired: 1 in]
            n154 = Index Array(array=w304, index (col)=6) -> (element=w306:dbl[])  [unwired: 1 in]
            n155 = Bundle(w312, w311, w310, w309, w308, w307, w306) -> ()  [unwired: 1 in, 1 out]
            n156 = Write to Binary File(file (use dialog)=w341, data=w304, 5:TRUE ("prepend array or string size? (T)")) -> (refnum out=w339:refnum<file>)  [unwired: 3 in, 2 out]
            n157 = local write "Save Indicator"(TRUE) -> ()
            n158 = Close File(refnum=w339) -> ()  [unwired: 1 in, 2 out]
          }
          frame 5 {
            n159 = property on="DATA Filename" class="Str"() -> ("Value"=w362:string)  [unwired: 2 in, 2 out]
            n160 = Concatenate Strings(w362, "_Decay.txt") -> (w366:string)
            n161 = Concatenate Strings(w362, "_Decay.acq") -> (w360:string)
            n162 = property on="Data Directory" class="Path"() -> ("Value"=w359:path)  [unwired: 2 in, 2 out]
            n163 = Build Path(base path=w359, name or relative path=w360) -> (appended path=w358:path)
            n164 = Build Path(base path=w359, name or relative path=w366) -> (appended path=w365:path)
            n165 = Open/Create/Replace File(file path (use dialog)=w358, operation (0:open)=T1."create") -> (refnum out=w364:refnum<file>)  [unwired: 4 in, 2 out]
            n166 = Build Array(w368, w367) -> (w355:dbl[][])
            n167 = Transpose 2D Array(2D array=w355) -> (transposed array=w354:dbl[][])
            n168 = Write to Binary File(file (use dialog)=w364, data=w354, 5:FALSE ("prepend array or string size? (T)")) -> (refnum out=w363:refnum<file>)  [unwired: 3 in, 2 out]
            n169 = call-poly <vilib>:"Write To Spreadsheet File.vi"("format (%.3f)"="%e", "2D data"=w354, "file path (dialog if empty)"=w365) -> ()  [unwired: 5 in, 1 out]
            n170 = Close File(refnum=w363) -> ()  [unwired: 1 in, 2 out]
          }
          frame 6 {
            (unwired) 100000
            w375 = 0.0
            w397 = 10123 items=["Finite Samples"=10178, "Continuous Samples"=10123] ("sample mode")
            w401 = T2 3 items=["no dialog", "OK message", "continue or stop message", "OK message + warnings", "continue/stop + warnings"] ("type of dialog (OK msg:1)")
            w405 = 10123 items=["Finite Samples"=10178, "Continuous Samples"=10123, "Hardware Timed Single Point"=12522] ("sample mode")
            n171 = call-poly <vilib>:"DAQmx Create Virtual Channel.vi"("maximum value"=10.0 ("maximum value 2"), "minimum value"=-10.0 ("minimum value 2"), "physical channels"=tag "Dev1/ao1" ("physical channels 2")) -> ("task out"=w407:refnum<k21>, "error out"=w406:errorcluster)  [unwired: 11 in]
            n172 = call-poly <vilib>:"DAQmx Create Virtual Channel.vi"("maximum value"=10.0 ("Maximum Value 2"), "minimum value"=-10.0 ("Minimum Value 2"), "physical channels"=tag "Dev1/ai0" ("Physical Channel 2")) -> ("task out"=w395:refnum<k21>, "error out"=w396:errorcluster)  [unwired: 11 in]
            n173 = call-poly <vilib>:"DAQmx Timing.vi"("task/channels in"=w395, "sample mode"=w397, "samples per channel"=2, "rate"=5000.0 ("Rate 2"), "error in"=w396) -> ("task out"=w391:refnum<k21>, "error out"=w390:errorcluster)  [unwired: 9 in]
            n174 = call-poly <vilib>:"DAQmx Timing.vi"("task/channels in"=w407, "sample mode"=w405, "rate"=5000, "error in"=w406) -> ("task out"=w404:refnum<k21>, "error out"=w403:errorcluster)  [unwired: 10 in]
            n175 = property class="DAQmx Timing" props=["Sample Clock:Rate"](reference=w391, error in=w390) -> (reference out=w389:refnum<k21>, error out=w388:errorcluster)  [unwired: 1 out]
            n176 = call <vilib>:"DAQmx Start Task.vi"("task/channels in"=w404, "error in"=w403) -> ("task out"=w402:refnum<k21>, "error out"=w384:errorcluster)  [unwired: 12 in]
            n177 = call "Get Terminal Name with Device Prefix.vi"("error in (no error)"=w388, "Local Terminal Name"="ai/StartTrigger" ("terminal"), "task/channels in"=w389) -> ("error out"=w372:errorcluster, "task out"=w373:refnum<k21>)  [unwired: 6 in, 1 out]
            n178 = property on="Waveform Chart" class="WFChart (strict)"("Visible"=TRUE) -> ()  [unwired: 2 in, 2 out]
            n179 = call <vilib>:"DAQmx Start Task.vi"("task/channels in"=w373, "error in"=w372) -> ("task out"=w382:refnum<k21>, "error out"=w386:errorcluster)  [unwired: 12 in]
            n180 = Initialize Array(w375, w375) -> ()  [unwired: 1 out]
            n181 = while {
              tunnel: w402 -> [w433]
              tunnel: w386 -> [w432]
              tunnel: w384 -> [w431]
              tunnel: ["Analog Ouyput 1"] -> w383
              tunnel: w382 -> [w430]
              tunnel: [w429] -> w381
              tunnel: [w428] -> w380
              tunnel: [w427] -> w378
              tunnel: [w421] -> w376
              stop <- w419 stop-if-true
              n182 = call-poly <vilib>:"DAQmx Read.vi"("task/channels in"=w430, "error in"=w432) -> ("task out"=w421:refnum<k21>, "data"=w418:dbl, "error out"=w427:errorcluster)  [unwired: 11 in]
              "Waveform Chart" <- w418
              n183 = call-poly <vilib>:"DAQmx Write.vi"("task/channels in"=w433, "data"="Analog Ouyput 1", "timeout"=0.1 ("Wirite Timeout"), "error in"=w431) -> ("task out"=w429:refnum<k21>, "error out"=w428:errorcluster)  [unwired: 9 in, 1 out]
              n184 = local read "Manual Z"() -> (w417:bool)
              n185 = Build Array("Analog Ouyput 1") -> (w425:dbl[])
              n186 = Build Array(w418) -> (w424:dbl[])
              n187 = Build Array(w424, w425) -> (w423:dbl[][])
              n188 = Not(x=w417) -> (.not. x?=w420:bool)
              n189 = Transpose 2D Array(2D array=w423) -> ()  [unwired: 1 out]
              n190 = Compound Arithmetic op=OR(TRUE ("value"), TRUE ("value"), w420) -> (w419:bool)
            }
            n191 = call <vilib>:"DAQmx Clear Task.vi"("task in"=w381, "error in"=w380) -> ("error out"=w379:errorcluster)  [unwired: 13 in]
            n192 = call <vilib>:"DAQmx Clear Task.vi"("task in"=w376, "error in"=w378) -> ("error out"=w377:errorcluster)  [unwired: 13 in]
            n193 = Merge Errors(w377, w379) -> (w385:errorcluster)
            n194 = call <vilib>:"General Error Handler.vi"("type of dialog (OK msg:1)"=w401, "error in (no error)"=w385) -> ()  [unwired: 9 in, 5 out]
          }
          frame 7 {
            w437 = 0.0
            w458 = T2 3 items=["no dialog", "OK message", "continue or stop message", "OK message + warnings", "continue/stop + warnings"] ("type of dialog (OK msg:1)")
            w473 = 10123 items=["Finite Samples"=10178, "Continuous Samples"=10123] ("sample mode")
            w467 = 10123 items=["Finite Samples"=10178, "Continuous Samples"=10123] ("sample mode")
            n195 = call-poly <vilib>:"DAQmx Create Virtual Channel.vi"("maximum value"=10.0 ("maximum value 2"), "minimum value"=-10.0 ("minimum value 2"), "physical channels"=tag "Dev1/ao1" ("physical channels 2")) -> ("task out"=w474:refnum<k21>, "error out"=w475:errorcluster)  [unwired: 11 in]
            n196 = call-poly <vilib>:"DAQmx Create Virtual Channel.vi"("maximum value"=10.0 ("Maximum Value 2"), "minimum value"=-10.0 ("Minimum Value 2"), "physical channels"=tag "Dev1/ai0" ("Physical Channel 2")) -> ("task out"=w469:refnum<k21>, "error out"=w468:errorcluster)  [unwired: 11 in]
            n197 = call-poly <vilib>:"DAQmx Timing.vi"("task/channels in"=w474, "sample mode"=w473, "rate"=10000.0 ("rate 2"), "error in"=w475) -> ("task out"=w482:refnum<k21>, "error out"=w483:errorcluster)  [unwired: 10 in]
            n198 = call-poly <vilib>:"DAQmx Timing.vi"("task/channels in"=w469, "sample mode"=w467, "rate"=10000.0 ("Rate 2"), "error in"=w468) -> ("task out"=w485:refnum<k21>, "error out"=w486:errorcluster)  [unwired: 10 in]
            n199 = property class="DAQmx Timing" props=["Sample Clock:Rate"](reference=w482, error in=w483) -> (reference out=w481:refnum<k21>, error out=w484:errorcluster)  [unwired: 1 out]
            n200 = property class="DAQmx Timing" props=["Sample Clock:Rate"](reference=w485, error in=w486) -> (reference out=w487:refnum<k21>, error out=w488:errorcluster)  [unwired: 1 out]
            n201 = call "Get Terminal Name with Device Prefix.vi"("error in (no error)"=w488, "Local Terminal Name"="ai/StartTrigger" ("terminal"), "task/channels in"=w487) -> ("error out"=w456:errorcluster, "Terminal Name with Device Prefix"=w480:tag, "task out"=w454:refnum<k21>)  [unwired: 6 in]
            n202 = call-poly <vilib>:"DAQmx Trigger.vi"("task/channels in"=w481, "source"=w480, "error in"=w484) -> ("task out"=w449:refnum<k21>, "error out"=w446:errorcluster)  [unwired: 11 in]
            n203 = Initialize Array(0.0, "Step Length") -> (w452:dbl[])
            n204 = call <vilib>:"DAQmx Start Task.vi"("task/channels in"=w454, "error in"=w456) -> ("task out"=w453:refnum<k21>, "error out"=w455:errorcluster)  [unwired: 12 in]
            n205 = call <vilib>:"DAQmx Start Task.vi"("task/channels in"=w449, "error in"=w446) -> ("task out"=w448:refnum<k21>, "error out"=w447:errorcluster)  [unwired: 12 in]
            n206 = Initialize Array(w437, w437) -> (w436:dbl[])
            n207 = while {
              tunnel: w453 -> [w509]
              tunnel: w455 -> [w508]
              tunnel: w448 -> [w507]
              tunnel: w447 -> [w506]
              tunnel: [w505] -> w464
              tunnel: [w504] -> w463
              tunnel: [w503] -> w461
              tunnel: [w502] -> w459
              shift-right: [w500] -> _
              shift-left: w452 -> [w501]
              tunnel: w444 -> [w498]
              shift-right: [w497] -> _
              shift-left: 1 -> [w496]
              shift-right: [w495] -> w440
              shift-left: w445 -> [w499]
              shift-right: [w493] -> w439
              shift-left: w436 -> [w494]
              shift-right: [w491] -> w438
              shift-left: w436 -> [w492]
              tunnel: [w489] -> w435
              stop <- w489 stop-if-true
              n208 = stacked-sequence {
                seq-local: [w511 _] -> [_ w551]
                tunnel: w509 -> [w542 _]
                tunnel: w508 -> [w541 _]
                tunnel: w507 -> [_ w559]
                tunnel: w506 -> [_ w558]
                tunnel: [w539 _] -> w505
                tunnel: [w540 _] -> w504
                tunnel: [_ w556] -> w503
                tunnel: [_ w557] -> w502
                tunnel: w501 -> [w536 w543]
                tunnel: [w519 _] -> w500
                tunnel: [w512 _] -> w489
                tunnel: w499 -> [_ w555]
                tunnel: w498 -> [_ w554]
                tunnel: [_ w553] -> w497
                tunnel: w496 -> [w528 w552]
                tunnel: "Ramp Rate" -> [_ w550]
                tunnel: [_ w548] -> _
                tunnel: [_ w548] -> w495
                tunnel: w494 -> [_ w547]
                tunnel: [_ w546] -> w493
                tunnel: w492 -> [_ w545]
                tunnel: [_ w544] -> w491
                frame #0 {
                  n209 = call-poly <vilib>:"DAQmx Read.vi"("task/channels in"=w542, "error in"=w541) -> ("task out"=w539:refnum<k21>, "data"=w510:dbl, "error out"=w540:errorcluster)  [unwired: 11 in]
                  n210 = Absolute Value(x=w510) -> (abs(x)=w511:dbl)
                  n211 = Insert Into Array(array=w536, index=0, new element=w511) -> (w537:dbl[])
                  n212 = local write "Waveform Chart"(w511) -> ()
                  n213 = Delete From Array(array=w537, length=1) -> (array with subset deleted=w519:dbl[])  [unwired: 1 in, 1 out]
                  n214 = Array Size(array=w519) -> (size(s)=w529:i32)
                  n215 = Decrement(x=w529) -> (x-1=w520:i32)
                  n216 = Index Array(array=w519, index=w520) -> (element=w522:dbl)
                  "element" <- w522
                  n217 = Index Array(array=w519, index=0) -> (element=w524:dbl)
                  n218 = Less?(x=w519, y="Step Max") -> (x < y?=w534:bool[])
                  n219 = Greater?(x=w519, y="Step Min") -> (0:w533:bool[])
                  n220 = Greater?(x="Step Min", y=w522) -> ()  [unwired: 1 out]
                  n221 = And Array Elements(Boolean array=w534) -> (logical AND=w518:bool)
                  n222 = And Array Elements(Boolean array=w533) -> (logical AND=w517:bool)
                  n223 = Less?(x="Step Max", y=w524) -> ()  [unwired: 1 out]
                  n224 = local read "Tapping"() -> (w514:bool)
                  n225 = And(x=w518, y=w517) -> (x .and. y?=w532:bool)
                  n226 = Equal?(x=w528, y=1) -> (x = y?=w526:bool)
                  n227 = Equal?(x=w528, y=2) -> (x = y?=w525:bool)
                  n228 = Or(x=w526, y=w525) -> (x .or. y?=w516:bool)
                  n229 = Not(x=w514) -> (.not. x?=w513:bool)
                  n230 = Compound Arithmetic op=AND(w532, w516) -> (w515:bool)
                  "Tapping Stop" <- w515
                  n231 = Or(x=w515, y=w513) -> (x .or. y?=w512:bool)
                }
                frame #1 {
                  n232 = case shown="1, Default" w552 {
                    tunnel: [w567 w590 w611 w637] -> w548
                    tunnel: w555 -> [w580 w592 w622 w634]
                    tunnel: [w575 w591 w616 w633] -> w553
                    tunnel: w551 -> [w566 _ w621 _]
                    tunnel: w550 -> [w581 w595 w623 w632]
                    tunnel: w547 -> [w571 w589 w610 _]
                    tunnel: [w573 w589 w610 w630] -> w546
                    tunnel: w545 -> [w565 w588 w609 _]
                    tunnel: [w572 w588 w609 w630] -> w544
                    tunnel: w543 -> [w564 _ _ _]
                    frame 1, Default {
                      w569 = -10
                      # "Breaking the contact"
                      n233 = Divide(x=w581, y=15.13) -> (x/y=w585:dbl)
                      n234 = Array Subset(array=w564, index=0, length=10) -> (w561:dbl[])
                      n235 = Divide(x=20, y=32768) -> (x/y=w582:dbl)
                      n236 = call-poly <vilib>:"Mean.vi"("X"=w561) -> ("mean"=w560:dbl)  [unwired: 1 out]
                      "mean" <- w560
                      n237 = Multiply(x=w582, y=w585) -> (x*y=w587:dbl)
                      n238 = Subtract(x=w580, y=w587) -> (x-y=w568:dbl)
                      n239 = Less?(x=w560, y="Min Current") -> (x < y?=w578:bool)
                      n240 = Select(t=2, s=w578, f=1) -> (s? t:f=w575:i32)
                      n241 = Build Array (concatenate)(w568, w571) -> (w573:dbl[])
                      n242 = Build Array (concatenate)(w566, w565) -> (w572:dbl[])
                      n243 = Less?(x=w568, y=w569) -> (x < y?=w570:bool)
                      n244 = local write "Contact Cycles"(0) -> ()
                      n245 = Select(t=w569, s=w570, f=w568) -> (s? t:f=w567:dbl)
                    }
                    frame 2 {
                      w607 = 10
                      # "Break contact cycles after current = 0"
                      n246 = Divide(x=w595, y=15.13) -> (x/y=w603:dbl)
                      n247 = local read "Contact Cycles"() -> (w594:i32)
                      n248 = Divide(x=20, y=32768) -> (x/y=w596:dbl)
                      n249 = Multiply(x=w596, y=w603) -> (x*y=w605:dbl)
                      n250 = Subtract(x=w592, y=w605) -> (x-y=w597:dbl)
                      n251 = Increment(x=w594) -> (x+1=w593:i32)
                      n252 = Less?(x=w597, y=w607) -> (x < y?=w606:bool)
                      n253 = Select(t=w597, s=w606, f=w607) -> (s? t:f=w590:dbl)
                      n254 = Less Or Equal?(x="Break Contact", y=w593) -> (x <= y?=w600:bool)
                      n255 = local write "Contact Cycles"(w593) -> ()
                      n256 = Select(t=3, s=w600, f=2) -> (s? t:f=w591:i32)
                    }
                    frame 3 {
                      w614 = 10
                      # "Making contact"
                      n257 = Divide(x=w623, y=15.13) -> (x/y=w627:dbl)
                      n258 = Divide(x=20, y=32768) -> (x/y=w624:dbl)
                      n259 = Multiply(x=w624, y=w627) -> (x*y=w629:dbl)
                      n260 = Add(x=w622, y=w629) -> (x+y=w612:dbl)
                      n261 = Greater?(x=w621, y="Max Current") -> (0:w619:bool)
                      n262 = Select(t=4, s=w619, f=3) -> (s? t:f=w616:i32)
                      n263 = local write "Contact Cycles"(0) -> ()
                      n264 = Less?(x=w612, y=w614) -> (x < y?=w613:bool)
                      n265 = Select(t=w612, s=w613, f=w614) -> (s? t:f=w611:dbl)
                    }
                    frame 4 {
                      w631 = 0.0
                      w649 = 10
                      # "Make contact cycles after current saturation"
                      n266 = Divide(x=w632, y=15.13) -> (x/y=w645:dbl)
                      n267 = local read "Contact Cycles"() -> (w639:i32)
                      n268 = Divide(x=20, y=32768) -> (x/y=w635:dbl)
                      n269 = Multiply(x=w635, y=w645) -> (x*y=w647:dbl)
                      n270 = Add(x=w634, y=w647) -> (x+y=w636:dbl)
                      n271 = Increment(x=w639) -> (x+1=w638:i32)
                      n272 = Less?(x=w636, y=w649) -> (x < y?=w648:bool)
                      n273 = Select(t=w636, s=w648, f=w649) -> (s? t:f=w637:dbl)
                      n274 = Less Or Equal?(x="Make Contact", y=w638) -> (x <= y?=w642:bool)
                      n275 = local write "Contact Cycles"(w638) -> ()
                      n276 = Initialize Array(w631, w631) -> (w630:dbl[])
                      n277 = Select(t=1, s=w642, f=4) -> (s? t:f=w633:i32)
                    }
                  }
                  n278 = local write "Analog Ouyput 1"(w548) -> ()
                  n279 = Build Array(w554, w548) -> ()  [unwired: 1 out]
                  n280 = call-poly <vilib>:"DAQmx Write.vi"("task/channels in"=w559, "auto start"=TRUE, "data"=w548, "error in"=w558) -> ("task out"=w557:refnum<k21>, "error out"=w556:errorcluster)  [unwired: 9 in, 1 out]
                }
              }
              "Case" <- w497
            }
            n281 = call <vilib>:"DAQmx Clear Task.vi"("task in"=w459, "error in"=w461) -> ("error out"=w460:errorcluster)  [unwired: 13 in]
            n282 = Not(x=w435) -> (.not. x?=w434:bool)
            n283 = call <vilib>:"DAQmx Clear Task.vi"("task in"=w464, "error in"=w463) -> ("error out"=w462:errorcluster)  [unwired: 13 in]
            n284 = local write "Tapping"(w434) -> ()
            n285 = Merge Errors(w462, w460) -> (w457:errorcluster)
            n286 = call <vilib>:"General Error Handler.vi"("type of dialog (OK msg:1)"=w458, "error in (no error)"=w457) -> ()  [unwired: 9 in, 5 out]
          }
          frame 8 {
            w656 = 0.0
            w670 = T2 3 items=["no dialog", "OK message", "continue or stop message", "OK message + warnings", "continue/stop + warnings"] ("type of dialog (OK msg:1)")
            w683 = 10123 items=["Finite Samples"=10178, "Continuous Samples"=10123] ("sample mode")
            w677 = 10123 items=["Finite Samples"=10178, "Continuous Samples"=10123] ("sample mode")
            n287 = call-poly <vilib>:"DAQmx Create Virtual Channel.vi"("maximum value"=10.0 ("maximum value 2"), "minimum value"=-10.0 ("minimum value 2"), "physical channels"=tag "Dev1/ao0:1" ("physical channels 2")) -> ("task out"=w684:refnum<k21>, "error out"=w685:errorcluster)  [unwired: 11 in]
            n288 = call-poly <vilib>:"DAQmx Create Virtual Channel.vi"("maximum value"=10.0 ("Maximum Value 2"), "minimum value"=-10.0 ("Minimum Value 2"), "physical channels"=tag "Dev1/ai0" ("Physical Channel 2")) -> ("task out"=w679:refnum<k21>, "error out"=w678:errorcluster)  [unwired: 11 in]
            n289 = call-poly <vilib>:"DAQmx Timing.vi"("task/channels in"=w684, "sample mode"=w683, "rate"=10000.0 ("rate 2"), "error in"=w685) -> ("task out"=w692:refnum<k21>, "error out"=w693:errorcluster)  [unwired: 10 in]
            n290 = call-poly <vilib>:"DAQmx Timing.vi"("task/channels in"=w679, "sample mode"=w677, "rate"=10000.0 ("Rate 2"), "error in"=w678) -> ("task out"=w695:refnum<k21>, "error out"=w696:errorcluster)  [unwired: 10 in]
            n291 = property class="DAQmx Timing" props=["Sample Clock:Rate"](reference=w692, error in=w693) -> (reference out=w691:refnum<k21>, error out=w694:errorcluster)  [unwired: 1 out]
            n292 = property class="DAQmx Timing" props=["Sample Clock:Rate"](reference=w695, error in=w696) -> (reference out=w697:refnum<k21>, error out=w698:errorcluster)  [unwired: 1 out]
            n293 = call "Get Terminal Name with Device Prefix.vi"("error in (no error)"=w698, "Local Terminal Name"="ai/StartTrigger" ("terminal"), "task/channels in"=w697) -> ("error out"=w668:errorcluster, "Terminal Name with Device Prefix"=w690:tag, "task out"=w666:refnum<k21>)  [unwired: 6 in]
            n294 = call-poly <vilib>:"DAQmx Trigger.vi"("task/channels in"=w691, "source"=w690, "error in"=w694) -> ("task out"=w664:refnum<k21>, "error out"=w661:errorcluster)  [unwired: 11 in]
            n295 = call <vilib>:"DAQmx Start Task.vi"("task/channels in"=w666, "error in"=w668) -> ("task out"=w665:refnum<k21>, "error out"=w667:errorcluster)  [unwired: 12 in]
            n296 = call <vilib>:"DAQmx Start Task.vi"("task/channels in"=w664, "error in"=w661) -> ("task out"=w663:refnum<k21>, "error out"=w662:errorcluster)  [unwired: 12 in]
            n297 = Initialize Array(w656, w656) -> ()  [unwired: 1 out]
            n298 = while {
              tunnel: w665 -> [w733]
              tunnel: w667 -> [w732]
              tunnel: w663 -> [w722]
              tunnel: w662 -> [w721]
              tunnel: [w731] -> w674
              tunnel: [w730] -> w673
              shift-right: [w708] -> w657
              shift-left: w660 -> [w712]
              tunnel: [w720] -> w655
              tunnel: [w719] -> w654
              tunnel: w651 -> [w704]
              i -> [w718]
              stop <- w709 stop-if-true
              w716 = 5e-05
              n299 = Absolute Value(x="Setpoint") -> (abs(x)=w700:dbl)
              n300 = call-poly <vilib>:"DAQmx Read.vi"("task/channels in"=w733, "error in"=w732) -> ("task out"=w731:refnum<k21>, "data"=w703:dbl, "error out"=w730:errorcluster)  [unwired: 11 in]
              n301 = Absolute Value(x=w703) -> (abs(x)=w702:dbl)
              n302 = local read "Bias Offset Correct"() -> (w705:dbl)
              n303 = Bundle("Proportional Gain"="Proportional Gain", "Integral Gain"="Integral Gain", "Differential Gain"="Differential Gain") -> (w723:T3)  [unwired: 1 in]
              n304 = local write "Waveform Chart"(w703) -> ()
              n305 = Bundle(10, -10) -> (w727:cluster{i32, i32})  [unwired: 1 in]
              n306 = call-poly "PID.vi"("output range"=w727, "dt (s)"=w716, "PID gains"=w723, "process variable"=w702, "setpoint"=w700) -> ("output"=w715:dbl)  [unwired: 5 in, 1 out]
              n307 = Add(x=w704, y=w705) -> (x+y=w706:dbl)
              n308 = Less?(x=w718, y=1000) -> (x < y?=w713:bool)
              n309 = call-poly "PID Output Rate Limiter.vi"("reinitialize? (F)"=w713, "dt (s)"=w716, "output rate (EGU/min)"="Piezo Delta rate", "initial output"=w712, "input (controller output)"=w715) -> ("output"=w708:dbl)  [unwired: 3 in, 1 out]
              n310 = local write "Analog Ouyput 1"(w708) -> ()
              n311 = Build Array(w706, w708) -> (w707:dbl[])
              n312 = local read "PID"() -> (w710:bool)
              n313 = call-poly <vilib>:"DAQmx Write.vi"("task/channels in"=w722, "data"=w707, "error in"=w721) -> ("task out"=w720:refnum<k21>, "error out"=w719:errorcluster)  [unwired: 10 in, 1 out]
              n314 = Not(x=w710) -> (.not. x?=w711:bool)
              n315 = Compound Arithmetic op=OR(FALSE ("value"), w711) -> (w709:bool)
            }
            n316 = call <vilib>:"DAQmx Clear Task.vi"("task in"=w655, "error in"=w654) -> ("error out"=w671:errorcluster)  [unwired: 13 in]
            n317 = call <vilib>:"DAQmx Clear Task.vi"("task in"=w674, "error in"=w673) -> ("error out"=w672:errorcluster)  [unwired: 13 in]
            n318 = Merge Errors(w672, w671) -> (w669:errorcluster)
            n319 = call <vilib>:"General Error Handler.vi"("type of dialog (OK msg:1)"=w670, "error in (no error)"=w669) -> ()  [unwired: 9 in, 5 out]
          }
        }
      }
    }
  }
